vi "CheckRouteForSerialNumber.vi"(0 "class data in":refnum<class "CMESAPI.lvclass">, 5 "serialNumber":string, 7 "equipment":string, 9 "WorkorderNumber":string, 11 "error in (no error)":errorcluster) -> (4 "class data out":refnum<class "CMESAPI.lvclass">, 6 "Result":bool, 8 "resulting string":string, 15 "error out":errorcluster)   [LabVIEW 2020, in "Salcomp-MES.lvlib" / "CMESAPI.lvclass"]
uses:
  CMESAPI.lvclass
  CMESAPI.lvclass/CMESAPI.ctl
  E:/Git/Libraries/develop/CME-API/CMESAPI_Fw4.0_1.9.2/CMESAPI.dll
  CMESAPI_Fw4.0_1.9.2/CMESAPI.dll
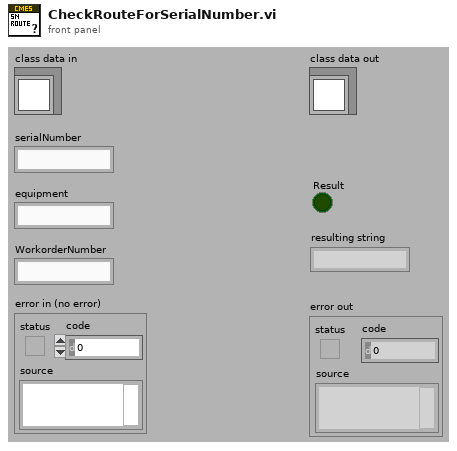
[diagram p1: front panel]
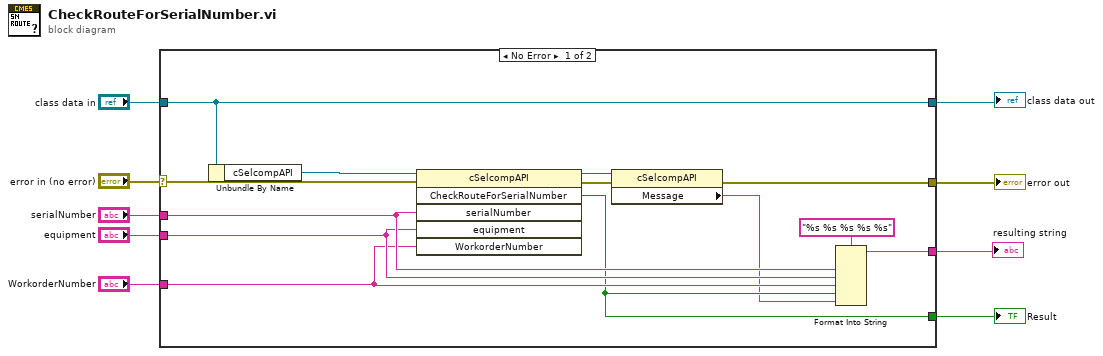
[diagram p0: block diagram]
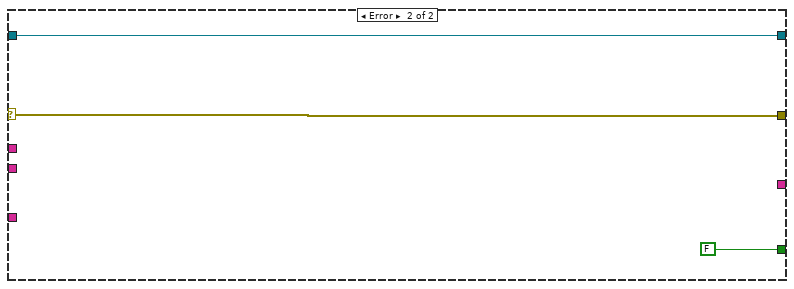
[diagram p2: hidden frame]
diagram:
  n1 = case shown="No Error" "error in (no error)" {
    selector: "error in (no error)" -> [w20 w25]
    tunnel: [w11 w25] -> w8
    tunnel: "class data in" -> [w22 w24]
    tunnel: [w22 w24] -> w6
    tunnel: "WorkorderNumber" -> [w15 _]
    tunnel: "equipment" -> [w16 _]
    tunnel: "serialNumber" -> [w17 _]
    tunnel: [w13 FALSE ("CheckRouteForSerialNumber")] -> w2
    tunnel: [w10 _] -> w1
    frame No Error {
      n2 = Unbundle By Name(w22) -> ("cSelcompAPI"=w21:refnum<k24>)
      n3 = invoke on="Invoke Node" class="cSelcompAPI" method="CheckRouteForSerialNumber"(reference=w21, error in=w20, "serialNumber"=w17, "equipment"=w16, "WorkorderNumber"=w15) -> (reference out=w18:refnum<k24>, error out=w19:errorcluster, "CheckRouteForSerialNumber"=w13:bool)  [unwired: 1 in, 3 out]
      n4 = property class="cSelcompAPI"(reference=w18, error in=w19) -> (error out=w11:errorcluster, "Message"=w12:string)  [unwired: 1 out]
      n5 = Format Into String(format string="%s %s %s %s %s", w17, w16, w15, w13, w12) -> (resulting string=w10:string)  [unwired: 2 in, 1 out]
    }
    frame Error {
    }
  }
  "error out" <- w8
  "class data out" <- w6
  "Result" <- w2
  "resulting string" <- w1
